vi "MPM_Set_Sweep_Speed.vi"(8 "error in (no error)":errorcluster, 10 "speed":dbl, 11 ".NET Reference in":refnum<k24>) -> (0 "error out":errorcluster, 3 "Reference out":refnum<k24>)   [LabVIEW 2017]
uses:
  D:/test/FULLband-sts/Fullband_Sample/DLL/InstrumentDLL.dll
  DLL/InstrumentDLL.dll
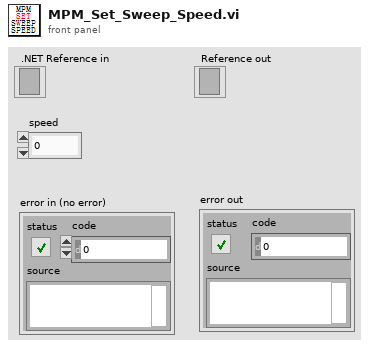
[diagram p1: front panel]
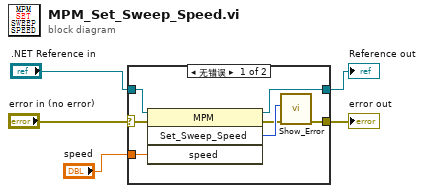
[diagram p0: block diagram]
diagram:
  n1 = case shown="无错误" "error in (no error)" {
    selector: "error in (no error)" -> [w9 w14]
    tunnel: [w10 w14] -> w5
    tunnel: ".NET Reference in" -> [w8 w13]
    tunnel: [w7 w13] -> w2
    tunnel: "speed" -> [w6 _]
    frame No Error {
      n2 = invoke class="MPM" method="Set_Sweep_Speed"(reference=w8, error in=w9, "speed"=w6) -> (reference out=w7:refnum<k24>, error out=w11:errorcluster, "Set_Sweep_Speed"=w12:i32)  [unwired: 1 in, 1 out]
      n3 = call "Show_Error.vi"("error in (no error)"=w11, "Error"=w12) -> ("error out"=w10:errorcluster)  [unwired: 9 in]
    }
    frame Error {
    }
  }
  "Reference out" <- w2
  "error out" <- w5
